vi "Add New Message.vi"(8 "error in (no error)":errorcluster, 11 "Node Ptr":u64 format="%.0x") -> (0 "error out":errorcluster)   [LabVIEW 2013, in "Instrument Addon System Explorer.lvlib"]
uses:
  Instrument Addon System Explorer.lvlib
  <vilib>/NI Veristand/Custom Device API/Custom Device Channel.ctl
  <vilib>/NI Veristand/Custom Device API/Custom Device Channel Type.ctl
  Shared/Constants.vi
  <vilib>/NI Veristand/Custom Device API/Custom Device API.lvlib
  Shared/Instrument Addon Shared.lvlib
panel:
  in  "Tag":string
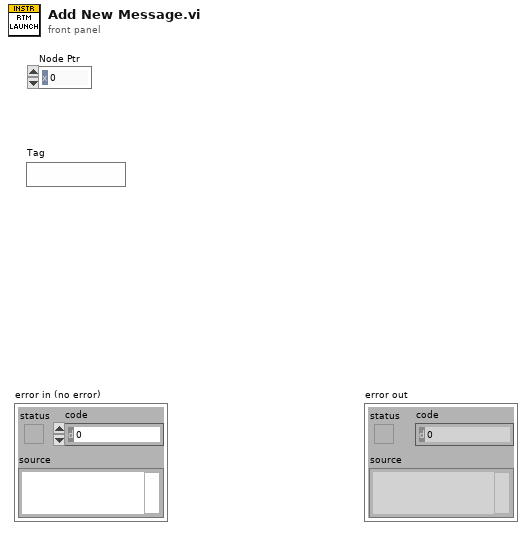
[diagram p1: front panel]
types:
  T1 = typedef "Custom Device API.lvlib/Custom Device Channel.ctl" = cluster{"Type":T2, "Units":string, "Default Value":dbl, "Faultable":bool, "Scalable":bool}
  T2 = typedef "Custom Device API.lvlib/Custom Device Channel Type.ctl" = enum16{"Input", "Output"}
  T3 = typedef "Custom Device API.lvlib/Custom Device Item Ref.ctl" = u64
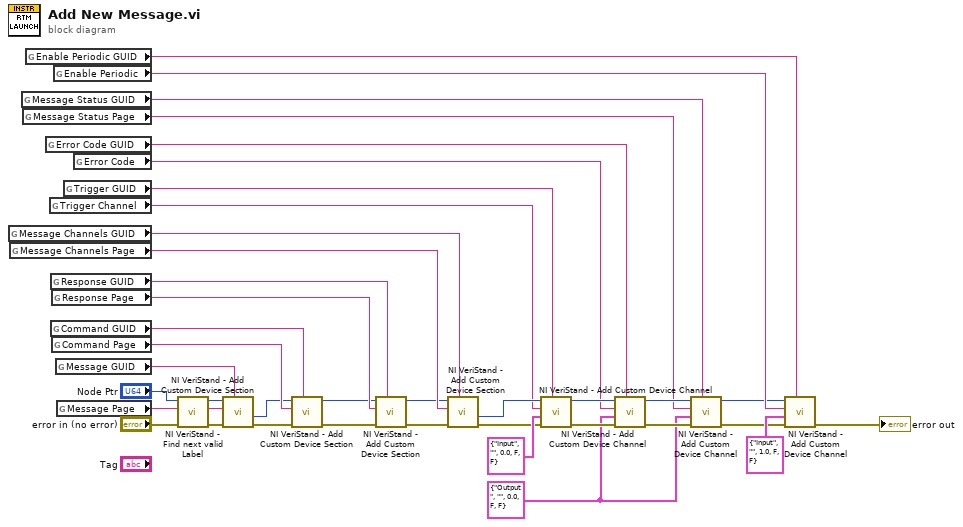
[diagram p0: block diagram]
diagram:
  w9 = T1 {"Type"=enum."Output", "Units"="", "Default Value"=0.0, "Faultable"=FALSE, "Scalable"=FALSE} ("Channel")
  n1 = global read "Constants.vi" "Message Channels GUID"() -> (w30:string)
  n2 = global read "Constants.vi" "Message Channels Page"() -> (w31:string)
  n3 = global read "Constants.vi" "Message Status GUID"() -> (w8:string)
  n4 = global read "Constants.vi" "Message Status Page"() -> (w7:string)
  n5 = global read "Constants.vi" "Enable Periodic GUID"() -> (w6:string)
  n6 = global read "Constants.vi" "Error Code GUID"() -> (w23:string)
  n7 = global read "Constants.vi" "Trigger Channel"() -> (w26:string)
  n8 = global read "Constants.vi" "Response GUID"() -> (w20:string)
  n9 = global read "Constants.vi" "Command GUID"() -> (w19:string)
  n10 = global read "Constants.vi" "Response Page"() -> (w21:string)
  n11 = global read "Constants.vi" "Command Page"() -> (w18:string)
  n12 = global read "Constants.vi" "Enable Periodic"() -> (w5:string)
  n13 = global read "Constants.vi" "Message GUID"() -> (w32:string)
  n14 = global read "Constants.vi" "Message Page"() -> (w33:string)
  n15 = global read "Constants.vi" "Trigger GUID"() -> (w27:string)
  n16 = global read "Constants.vi" "Error Code"() -> (w22:string)
  n17 = call <vilib>:"NI VeriStand - Find next valid Label.vi"("error in (no error)"="error in (no error)", "Label"=w33, "Item Ref in"="Node Ptr") -> ("error out"=w37:errorcluster, "Label out"=w36:string, "Item Ref out"=w35:T3)  [unwired: 4 in, 2 out]
  n18 = call <vilib>:"NI VeriStand - Add Custom Device Section.vi"("GUID (Default Section)"=w32, "error in (no error)"=w37, "Section Name"=w36, "Parent Ref in"=w35) -> ("error out"=w14:errorcluster, "Section Ptr"=w15:T3)  [unwired: 4 in, 2 out]
  n19 = call <vilib>:"NI VeriStand - Add Custom Device Section.vi"("GUID (Default Section)"=w19, "error in (no error)"=w14, "Section Name"=w18, "Parent Ref in"=w15) -> ("error out"=w17:errorcluster, "Parent Ref out"=w16:T3)  [unwired: 4 in, 2 out]
  n20 = call <vilib>:"NI VeriStand - Add Custom Device Section.vi"("GUID (Default Section)"=w20, "error in (no error)"=w17, "Section Name"=w21, "Parent Ref in"=w16) -> ("error out"=w13:errorcluster, "Parent Ref out"=w12:T3)  [unwired: 4 in, 2 out]
  n21 = call <vilib>:"NI VeriStand - Add Custom Device Section.vi"("GUID (Default Section)"=w30, "error in (no error)"=w13, "Section Name"=w31, "Parent Ref in"=w12) -> ("error out"=w29:errorcluster, "Section Ptr"=w28:T3)  [unwired: 4 in, 2 out]
  n22 = call <vilib>:"NI VeriStand - Add Custom Device Channel.vi"("GUID (Default Channel)"=w27, "error in (no error)"=w29, "Channel"=T1 {"Type"=enum."Input", "Units"="", "Default Value"=0.0, "Faultable"=FALSE, "Scalable"=FALSE}, "Channel Name"=w26, "Parent Ref in"=w28) -> ("error out"=w25:errorcluster, "Parent Ref out"=w24:T3)  [unwired: 3 in, 2 out]
  n23 = call <vilib>:"NI VeriStand - Add Custom Device Channel.vi"("GUID (Default Channel)"=w23, "error in (no error)"=w25, "Channel"=w9, "Channel Name"=w22, "Parent Ref in"=w24) -> ("error out"=w11:errorcluster, "Parent Ref out"=w10:T3)  [unwired: 3 in, 2 out]
  n24 = call <vilib>:"NI VeriStand - Add Custom Device Channel.vi"("GUID (Default Channel)"=w8, "error in (no error)"=w11, "Channel"=w9, "Channel Name"=w7, "Parent Ref in"=w10) -> ("error out"=w3:errorcluster, "Parent Ref out"=w2:T3)  [unwired: 3 in, 2 out]
  n25 = call <vilib>:"NI VeriStand - Add Custom Device Channel.vi"("GUID (Default Channel)"=w6, "error in (no error)"=w3, "Channel"=T1 {"Type"=enum."Input", "Units"="", "Default Value"=1.0, "Faultable"=FALSE, "Scalable"=FALSE}, "Channel Name"=w5, "Parent Ref in"=w2) -> ("error out"=→"error out":errorcluster)  [unwired: 3 in, 3 out]
